vi "equ2hor.vi"(4 "deltat [TT-UT1]":dbl[unit], 5 "TimeStamp [UT1]":timestamp format="%<%H:%M:%S%6u\n%Y/%m/%d>T", 6 "error in (no error)":errorcluster, 7 "on_surface":T1={"latitude"=0.3460406188465066, "longitude"=-2.713521559899553, "height"=4123.0, "temperature"=0.0, "pressure"=0.0} {"longitude" format="%_10g"; "latitude" format="%_10g"}, 9 "ra/dec":cluster{"ra":dbl[unit], "dec":dbl[unit]} {"dec" format="%_10g"; "ra" format="%_10g"}) -> (0 "error out":errorcluster, 1 "ra/dec (refraction)":cluster{"ra":dbl[unit], "dec":dbl[unit]} {"dec" format="%_10g"; "ra" format="%_10g"}, 3 "az/zd":cluster{"az":dbl[unit], "zd":dbl[unit]})   [LabVIEW 2009]
uses:
  Controls/SiteInformation.ctl
  lib/novas-dll.dll
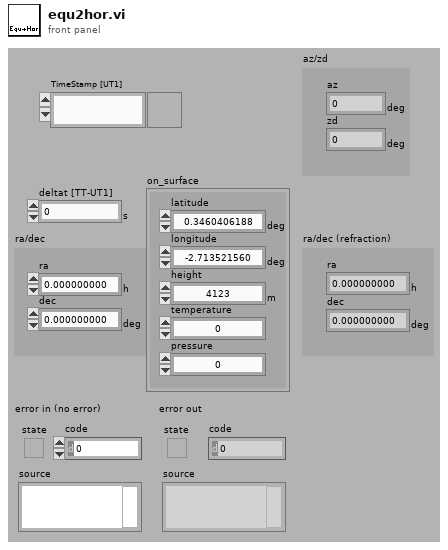
[diagram p1: front panel]
types:
  T1 = typedef "SiteInformation.ctl" = cluster{"latitude":dbl[unit], "longitude":dbl[unit], "height":dbl[unit], "temperature":dbl, "pressure":dbl}
  T2 = cluster{"latitude":dbl, "longitude":dbl, "height":dbl, "temperature":dbl, "pressure":dbl}
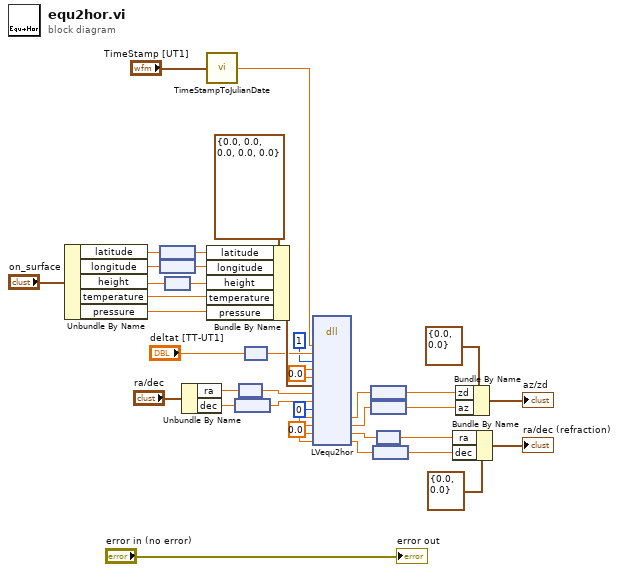
[diagram p0: block diagram]
diagram:
  w29 = 0.0 ("x")
  w36 = 0.0 ("x")
  n1 = Unbundle By Name("on_surface") -> ("latitude"=w25:dbl[unit], "longitude"=w24:dbl[unit], "height"=w23:dbl[unit], "temperature"=w22:dbl, "pressure"=w21:dbl)
  n2 = node(w25) -> (w18:dbl)
  n3 = node(w24) -> (w19:dbl)
  n4 = node(w23) -> (w20:dbl)
  n5 = Unbundle By Name("ra/dec") -> ("ra"=w34:dbl[unit], "dec"=w33:dbl[unit])
  n6 = call "TimeStampToJulianDate.vi"("TimeStamp [UT]"="TimeStamp [UT1]") -> ("JulianDay"=w3:ext)
  n7 = Bundle By Name(cluster=T2 {"latitude"=0.0, "longitude"=0.0, "height"=0.0, "temperature"=0.0, "pressure"=0.0} ("site_info"), "latitude"=w18, "longitude"=w19, "height"=w20, "temperature"=w22, "pressure"=w21) -> (w16:T2)
  n8 = node(w33) -> (w31:dbl)
  n9 = node(w34) -> (w32:dbl)
  n10 = node("deltat [TT-UT1]") -> (w15:dbl)
  n11 = dll-call lib="C:/OhanaOS/Instruments/Novas/lib/novas-dll.dll" fn="LVequ2hor"("jd_ut1"=w3, "delta_t"=w15, "accuracy"=i16 1, "x"=w36, "y"=w36, "location"=w16, "ra"=w32, "dec"=w31, "ref_option"=i16 0, "zd"=w29, "az"=w29, "rar"=w29, "decr"=w29) -> ("zd"=w28:dbl, "az"=w27:dbl, "rar"=w4:dbl, "decr"=w10:dbl)  [unwired: 10 in, 5 out]
  n12 = node(w28) -> (w12:dbl[unit])
  n13 = node(w27) -> (w11:dbl[unit])
  n14 = node(w10) -> (w6:dbl[unit])
  n15 = node(w4) -> (w7:dbl[unit])
  n16 = Bundle By Name(cluster=cluster{"ra":dbl[unit], "dec":dbl[unit]} {"ra"=0.0, "dec"=0.0} ("ra/dec (refraction)"), "ra"=w7, "dec"=w6) -> (→"ra/dec (refraction)":cluster{"ra":dbl[unit], "dec":dbl[unit]})
  n17 = Bundle By Name(cluster=cluster{"az":dbl[unit], "zd":dbl[unit]} {"az"=0.0, "zd"=0.0} ("az/zd"), "zd"=w12, "az"=w11) -> (→"az/zd":cluster{"az":dbl[unit], "zd":dbl[unit]})
  "error out" <- "error in (no error)"
